vi "Read simulated adc.vi"(8 "error in (no error)":errorcluster, 9 "Canal":u8, 11 "Simulada in":refnum<class "Simulada.lvclass">) -> (0 "error out":errorcluster, 1 "Expected response":string, 3 "Simulada out":refnum<class "Simulada.lvclass">)   [LabVIEW 2020, in "Simulada.lvclass"]
uses:
  Simulada.lvclass
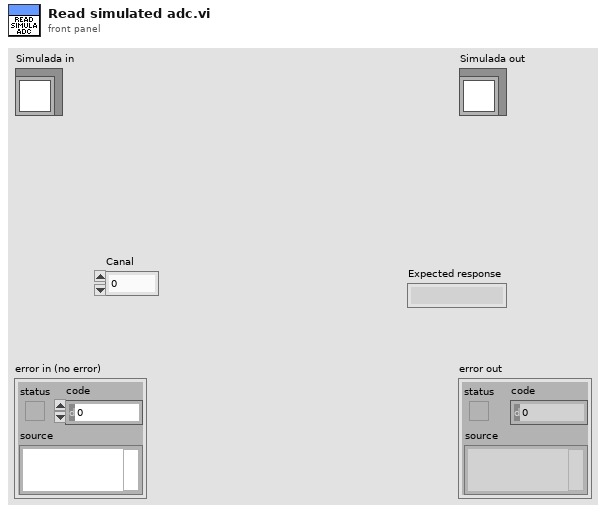
[diagram p1: front panel]
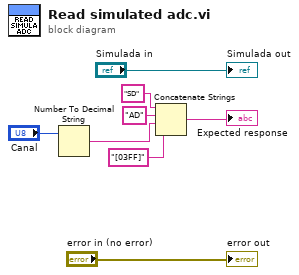
[diagram p0: block diagram]
diagram:
  n1 = Number To Decimal String(number="Canal") -> (decimal integer string=w3:string)  [unwired: 1 in]
  n2 = Concatenate Strings("SD" ("string"), "AD" ("string"), w3, "[03FF]" ("string")) -> (→"Expected response":string)
  "error out" <- "error in (no error)"
  "Simulada out" <- "Simulada in"
